vi "Comm_FGV(SubVI).vi"(7 "Enum":T1, 8 "error in (no error)":errorcluster) -> (0 "error out":errorcluster, 3 "Array":refnum<queue>[](array[refnum]))   [LabVIEW 2017, in "MainFrameLib.lvlib"]
uses:
  MainFrameLib.lvlib
  TypeDefs/FGV_Enum.ctl
  TypeDefs/DataCluster.ctl
  TypeDefs/Command_Enum.ctl
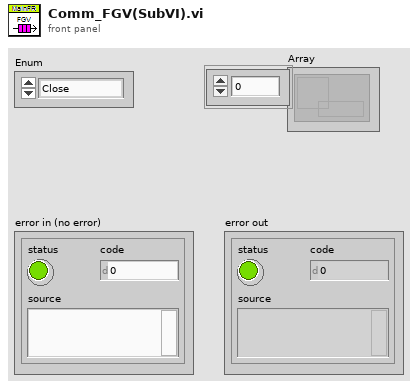
[diagram p1: front panel]
types:
  T1 = typedef "MainFrameLib.lvlib/FGV_Enum.ctl" = enum16{"Close", "GetRefs", "Initialize"}
  T2 = typedef "MainFrameLib.lvlib/DataCluster.ctl" = cluster{"Command":T3, "Data":variant}
  T3 = typedef "MainFrameLib.lvlib/Command_Enum.ctl" = enum16{"CheckSRLinks", "UpdateKCSColorCode", "StartLinkageCheck", "GetSRNotes", "DisplayAEStats", "InWork&Neglected", "RemapAENames", "ClearFolder", "UpdateReportsList", "ExcelReports", "TeamStats", "LoadReport", "WaitOnReport", "RequestReport", "Error", "Idle", "InitializeData", "ScreenPop", "Initialize", "UpdateCiscoAgentsView", "CancelRequests", "ClipboardCopy", "SaveNeglectedToFile", "Shutdown"}
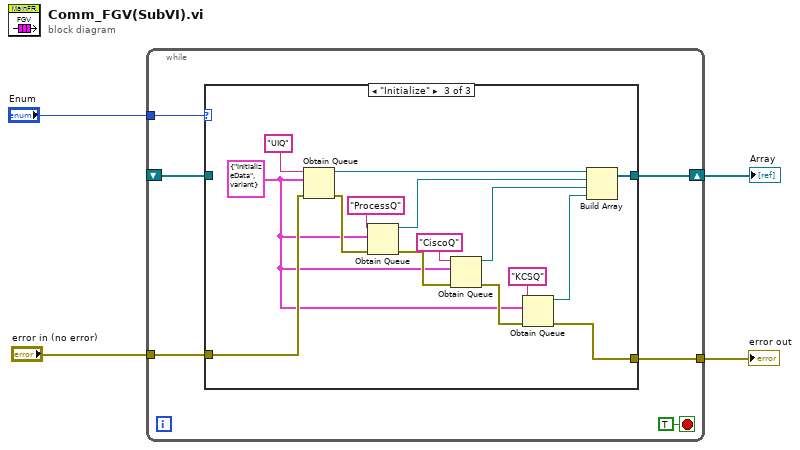
[diagram p0: block diagram]
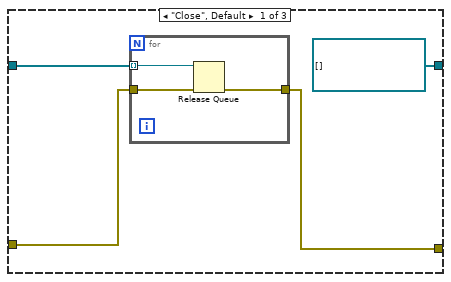
[diagram p2: hidden frame]
diagram:
  n1 = while {
    tunnel: "Enum" -> [w10]
    tunnel: "error in (no error)" -> [w8]
    tunnel: [w7] -> w4
    shift-right: [w6] -> w1
    shift-left: _ -> [w5]
    stop <- TRUE stop-if-true
    n2 = case shown="\"Initialize\"" w10 {
      tunnel: w8 -> [w13 w18 w32]
      tunnel: [w12 w18 w23] -> w7
      tunnel: [refnum<queue>[] [] w19 w28] -> w6
      tunnel: w5 -> [w14 w19 _]
      frame "Close", Default {
        n3 = for {
          tunnel: w14 -> [w17] mode=indexing
          tunnel: w13 -> [w16]
          tunnel: [w15] -> w12
          n4 = Release Queue(queue=w17, error in (no error)=w16) -> (error out=w15:errorcluster)  [unwired: 1 in, 2 out]
        }
      }
      frame "GetRefs" {
      }
      frame "Initialize" {
        w21 = T2 {"Command"=enum."InitializeData", "Data"=variant} ("Cluster")
        n5 = Obtain Queue(name (unnamed)="UIQ", element data type=w21, error in (no error)=w32) -> (queue out=w30:refnum<queue>, error out=w31:errorcluster)  [unwired: 2 in, 1 out]
        n6 = Obtain Queue(name (unnamed)="ProcessQ", element data type=w21, error in (no error)=w31) -> (queue out=w29:refnum<queue>, error out=w26:errorcluster)  [unwired: 2 in, 1 out]
        n7 = Obtain Queue(name (unnamed)="CiscoQ", element data type=w21, error in (no error)=w26) -> (queue out=w25:refnum<queue>, error out=w24:errorcluster)  [unwired: 2 in, 1 out]
        n8 = Obtain Queue(name (unnamed)="KCSQ", element data type=w21, error in (no error)=w24) -> (queue out=w22:refnum<queue>, error out=w23:errorcluster)  [unwired: 2 in, 1 out]
        n9 = Build Array(w30, w29, w25, w22) -> (w28:refnum<queue>[])
      }
    }
  }
  "error out" <- w4
  "Array" <- w1
